vi "displayDialog.vi"(0 "HB_Dialog in":refnum<class "HB_Dialog.lvclass">=refnum, 7 "Message":string, 11 "error in (no error)":errorcluster) -> (4 "HB_Dialog out":refnum<class "HB_Dialog.lvclass">, 8 "Button Index":i16, 15 "error out":errorcluster)   [LabVIEW 2009, in "HB_Inherance_Example.lvlib" / "HB_Dialog.lvclass"]
doc: "Static VI calling the protected dynamic dispatch VI. Sub classes must implement the display of the dialog."
uses:
  HB_Dialog.lvclass
  HB_TwoButtonDiolog/HB_TwoButtonDiolog.lvclass
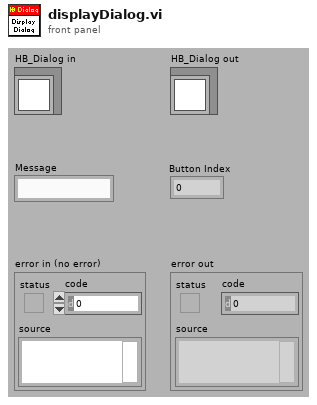
[diagram p1: front panel]
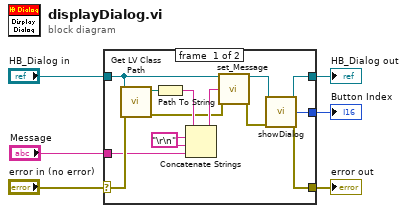
[diagram p0: block diagram]
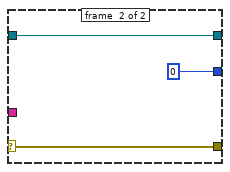
[diagram p2: hidden frame]
diagram:
  n1 = case shown="No Error" "error in (no error)" {
    selector: "error in (no error)" -> [w15 w22]
    tunnel: [w17 w22] -> w5
    tunnel: [w19 w21] -> w3
    tunnel: "HB_Dialog in" -> [w10 w21]
    tunnel: [w18 i16 0 ("Button Index")] -> w2
    tunnel: "Message" -> [w11 _]
    frame #0 {
      w7 = "\r\n"
      n2 = call <vilib>:"Get LV Class Path.vi"("error in (no error)"=w15, "object"=w10) -> ("error out"=w8:errorcluster, "class path"=w12:path)  [unwired: 8 in]
      n3 = Path To String(path=w12) -> (string=w13:string)
      n4 = Concatenate Strings(w13, w7, w7, w11) -> (w9:string)
      n5 = call "set_Message.vi"("HB_Dialog in"=w10, "Message"=w9, "error in (no error)"=w8) -> ("HB_Dialog out"=w16:refnum<class "HB_Dialog.lvclass">, "error out"=w14:errorcluster)  [unwired: 11 in]
      n6 = call-dynamic "showDialog.vi"("HB_Dialog in"=w16, "error in (no error)"=w14) -> ("HB_Dialog out"=w19:refnum<class "HB_Dialog.lvclass">, "Button Index"=w18:i16, "error out"=w17:errorcluster)  [unwired: 11 in]
    }
    frame #1 {
    }
  }
  "error out" <- w5
  "HB_Dialog out" <- w3
  "Button Index" <- w2
